vi "Test ZMQ RepReq.vi"() -> ()   [LabVIEW 2019, in "RemoteControl.ZMQ.lvclass"]
uses:
  <vilib>/addons/zeromq/socket_type.ctl
  RemoteControl.ZMQ.lvclass
  <vilib>/addons/zeromq/zmq_socket.lvclass
  <vilib>/addons/zeromq/zmq_context.lvclass
  <vilib>/addons/zeromq/zeromq.lvlib
panel:
  out "terminated":bool
  out "send multi":bool
  out "recv multi":bool
  out "error out":errorcluster
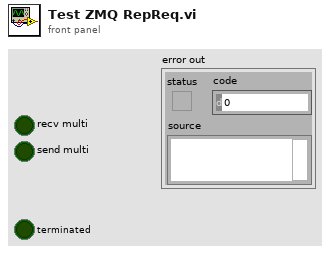
[diagram p1: front panel]
types:
  T1 = typedef "zeromq.lvlib/socket_type.ctl" = enum8{"ZMQ_PAIR", "ZMQ_PUB", "ZMQ_SUB", "ZMQ_REQ", "ZMQ_REP", "ZMQ_DEALER", "ZMQ_ROUTER", "ZMQ_PULL", "ZMQ_PUSH", "ZMQ_XPUB", "ZMQ_XSUB", "ZMQ_STREAM", "ZMQ_SERVER", "ZMQ_CLIENT", "ZMQ_RADIO", "ZMQ_DISH", "ZMQ_GATHER", "ZMQ_SCATTER", "ZMQ_DGRAM"}
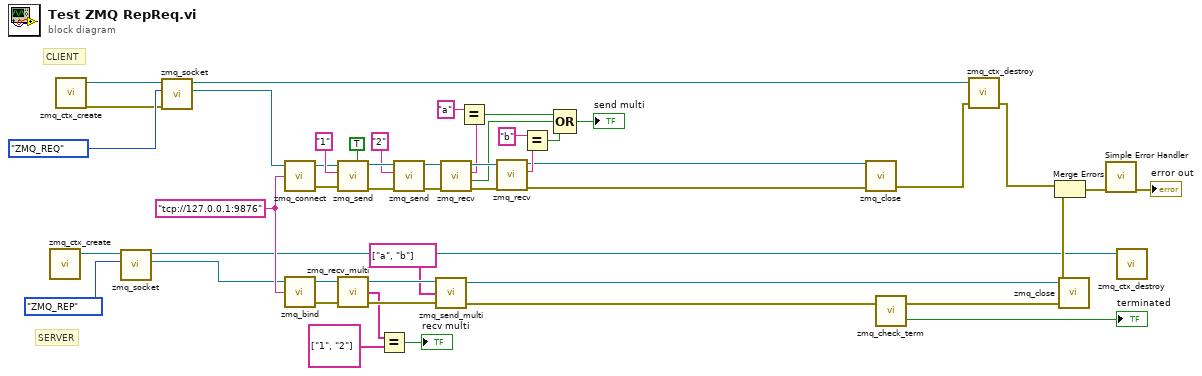
[diagram p0: block diagram]
diagram:
  w44 = "tcp://127.0.0.1:9876"
  # "SERVER"
  # "CLIENT"
  n1 = call <vilib>:"zmq_ctx_create.vi"() -> ("context out"=w2:refnum<class "zmq_context.lvclass">)  [unwired: 4 in, 1 out]
  n2 = call <vilib>:"zmq_ctx_create.vi"() -> ("error out"=w3:errorcluster, "context out"=w4:refnum<class "zmq_context.lvclass">)  [unwired: 4 in]
  n3 = call <vilib>:"zmq_socket.vi"("socket type"=socket_type."ZMQ_REP", "context in"=w2) -> ("socket out"=w11:refnum<class "zmq_socket.lvclass">, "context out"=w1:refnum<class "zmq_context.lvclass">)  [unwired: 3 in, 1 out]
  n4 = call <vilib>:"zmq_socket.vi"("error in"=w3, "socket type"=socket_type."ZMQ_REQ", "context in"=w4) -> ("socket out"=w12:refnum<class "zmq_socket.lvclass">, "context out"=w10:refnum<class "zmq_context.lvclass">)  [unwired: 2 in, 1 out]
  n5 = call <vilib>:"zmq_connect.vi"("endpoint"=w44, "socket in"=w12) -> ("error out"=w27:errorcluster, "socket out"=w28:refnum<class "zmq_socket.lvclass">)  [unwired: 2 in]
  n6 = call <vilib>:"zmq_bind.vi"("endpoint"=w44, "socket in"=w11) -> ("error out"=w29:errorcluster, "socket out"=w30:refnum<class "zmq_socket.lvclass">)  [unwired: 2 in]
  n7 = call <vilib>:"zmq_send.vi"("error in"=w27, "data"="1", "socket in"=w28, "more? (F)"=TRUE) -> ("error out"=w42:errorcluster, "socket out"=w46:refnum<class "zmq_socket.lvclass">)  [unwired: 3 in]
  n8 = call <vilib>:"zmq_recv_multi.vi"("error in"=w29, "socket in"=w30) -> ("error out"=w32:errorcluster, "parts"=w24:string[], "socket out"=w33:refnum<class "zmq_socket.lvclass">)  [unwired: 1 in]
  n9 = Equal?(x=w24, y=string[] ["1", "2"] ("12")) -> (x = y?=→"recv multi":bool)
  n10 = call <vilib>:"zmq_send.vi"("error in"=w42, "data"="2", "socket in"=w46) -> ("error out"=w35:errorcluster, "socket out"=w37:refnum<class "zmq_socket.lvclass">)  [unwired: 4 in]
  n11 = call <vilib>:"zmq_send_multi.vi"("error in"=w32, "parts"=string[] ["a", "b"], "socket in"=w33) -> ("error out"=w5:errorcluster, "socket out"=w6:refnum<class "zmq_socket.lvclass">)  [unwired: 1 in]
  n12 = call <vilib>:"zmq_recv.vi"("error in"=w35, "socket in"=w37) -> ("error out"=w34:errorcluster, "more?"=w16:bool, "data"=w21:string, "socket out"=w36:refnum<class "zmq_socket.lvclass">)  [unwired: 3 in, 1 out]
  n13 = Equal?(x="a" ("a"), y=w21) -> (x = y?=w18:bool)
  n14 = call <vilib>:"zmq_recv.vi"("error in"=w34, "socket in"=w36) -> ("error out"=w7:errorcluster, "data"=w20:string, "socket out"=w8:refnum<class "zmq_socket.lvclass">)  [unwired: 3 in, 2 out]
  n15 = Equal?(x="b" ("b"), y=w20) -> (x = y?=w17:bool)
  n16 = Compound Arithmetic op=OR(w18, w16, w17) -> (→"send multi":bool)
  n17 = call <vilib>:"zmq_close.vi"("error in"=w7, "socket"=w8) -> ("error out"=w26:errorcluster)  [unwired: 3 in]
  n18 = call <vilib>:"zmq_check_term.vi"("error in"=w5) -> ("term?"=→"terminated":bool, "error out"=w43:errorcluster)  [unwired: 1 in]
  n19 = call <vilib>:"zmq_ctx_destroy.vi"("error in"=w26, "context in"=w10) -> ("error out"=w41:errorcluster)  [unwired: 3 in]
  n20 = call <vilib>:"zmq_close.vi"("error in"=w43, "socket"=w6) -> ("error out"=w40:errorcluster)  [unwired: 3 in]
  n21 = Merge Errors(w41, w40) -> (w14:errorcluster)
  n22 = call <vilib>:"Simple Error Handler.vi"("error in (no error)"=w14) -> ("error out"=→"error out":errorcluster)  [unwired: 4 in, 4 out]
  n23 = call <vilib>:"zmq_ctx_destroy.vi"("context in"=w1) -> ()  [unwired: 4 in, 1 out]
